vi "Run Action_Do.vi"(8 "error in (no error)":errorcluster, 10 "Project Builder in":refnum<class "Project Builder.lvclass">, 11 "Run System Exec":refnum<class "Run System Exec.lvclass">) -> (0 "error out":errorcluster, 1 "Success?":bool, 3 "Report":refnum<class "Report Data.lvclass">)   [LabVIEW 2019, in "ProjectBuilder.lvlib" / "Run System Exec.lvclass"]
doc: "Run the action associated with the 'Project Action'-class.\n\nThis implementation runs System Exec.vi with the provided input."
uses:
  Run System Exec.lvclass
  Project Builder/Project Builder.lvclass
  System Exec Data/System Exec Data.lvclass
  Data/Report Data/Report Data.lvclass
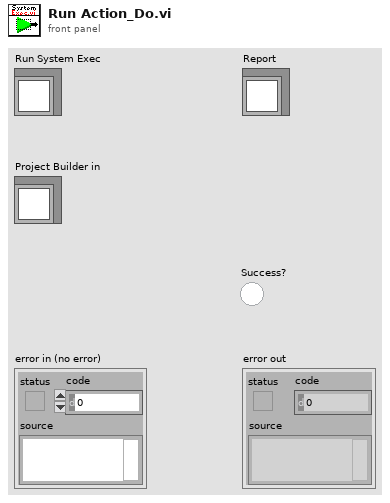
[diagram p1: front panel]
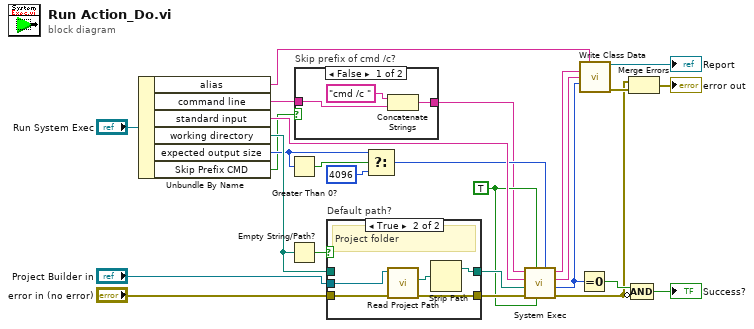
[diagram p0: block diagram]
diagram:
  w12 = TRUE ("wait until completion? (T)")
  n1 = Unbundle By Name("Run System Exec") -> ("alias"=w1:string, "command line"=w9:string, "standard input"=w25:string, "working directory"=w21:path, "expected output size"=w19:u32, "Skip Prefix CMD"=w11:bool)
  n2 = Greater Than 0?(x=w19) -> (x > 0?=w20:bool)
  n3 = Empty String/Path?(string/path=w21) -> (empty?=w23:bool)
  n4 = case "Skip prefix of cmd /c?" shown="False" w11 {
    tunnel: [w27 w30] -> w10
    tunnel: w9 -> [w28 w30]
    frame False {
      n5 = Concatenate Strings("cmd /c ", w28) -> (w27:string)
    }
    frame True {
    }
  }
  n6 = case "Default path?" shown="True" w23 {
    tunnel: "error in (no error)" -> [w31 w35]
    tunnel: [w32 w37] -> w22
    tunnel: w21 -> [w32 _]
    tunnel: [w31 w33] -> w16
    tunnel: "Project Builder in" -> [_ w36]
    frame False {
      # "Non default"
    }
    frame True {
      # "Project folder"
      n7 = call "Read Project Path.vi"("error in (no error)"=w35, "Project Builder in"=w36) -> ("error out"=w33:errorcluster, "Project Path"=w34:path)  [unwired: 7 in, 1 out]
      n8 = Strip Path(path=w34) -> (stripped path=w37:path)  [unwired: 1 out]
    }
  }
  n9 = Select(t=w19, s=w20, f=u32 4096 ("expected output size  (4096)")) -> (s? t:f=w17:u32)
  n10 = call <vilib>:"System Exec.vi"("expected output size  (4096)"=w17, "run minimized? (F)"=w12, "wait until completion? (T)"=w12, "error in (no error)"=w16, "working directory"=w22, "standard input"=w25, "command line"=w10) -> ("error out"=w3:errorcluster, "return code"=w5:i32, "standard error"=w6:string, "standard output"=w8:string)  [unwired: 1 in]
  n11 = Equal To 0?(x=w5) -> (x = 0?=w15:bool)
  n12 = call "Write Class Data.vi"("alias"=w1, "standard output"=w8, "standard error"=w6, "return code"=w5) -> ("System Exec Data out"=→"Report":refnum<class "System Exec Data.lvclass">, "error out"=w4:errorcluster)  [unwired: 10 in]
  n13 = Merge Errors(w3, w4) -> (→"error out":errorcluster)
  n14 = Compound Arithmetic op=AND(w15, invert w3) -> (→"Success?":bool)
